vi "Modbus_建立连接.vi"(8 "error in (no error)":errorcluster caption="错误输入（无错误）", 10 "Mod ID":i32, 11 "Mod":T1) -> (0 "error out":errorcluster caption="错误输出", 3 "Mod 2":T1)   [LabVIEW 2018]
uses:
  <vilib>/Modbus/master/Modbus Master.lvclass
  C:/Program Files (x86)/National Instruments/LabVIEW 2018/vi.lib/Modbus/subvis/Modbus API/Modbus API.lvclass
  <vilib>/Modbus/subvis/Modbus API/Modbus API.lvclass/Modbus API.ctl
  <vilib>/Modbus/subvis/Transmission Data Unit (ADU)/Transmission Data Unit/Transmission Data Unit.lvclass/Transmission Data Unit.ctl
  <vilib>/Modbus/master/Data Access/Read Timeout/Set Read Timeout.vi
  <vilib>/Modbus/master/Data Access/Write Timeout/Set Write Timeout.vi
  <vilib>/Modbus/master/Data Access/Unit ID/Set Unit ID Property.vi
  <vilib>/Modbus/subvis/Modbus API/Read Transmission Data Unit.vi
  <vilib>/Modbus/subvis/Modbus API/Write Transmission Data Unit.vi
  <vilib>/Modbus/subvis/Transmission Data Unit (ADU)/Transmission Data Unit/Data Access/timeouts/Write read operation timeout.vi
  <vilib>/Modbus/subvis/Transmission Data Unit (ADU)/Transmission Data Unit/Data Access/timeouts/Write write operation timeout.vi
  <vilib>/Modbus/subvis/Transmission Data Unit (ADU)/Transmission Data Unit/Data Access/Unit ID/Write Unit ID.vi
  <vilib>/Modbus/master/Create Master Instance (Serial).vi
  <vilib>/Modbus/master/Create Master Instance (TCP).vi
  <vilib>/Modbus/subvis/Transmission Data Unit (ADU)/Transmission Data Unit/Transmission Data Unit.lvclass
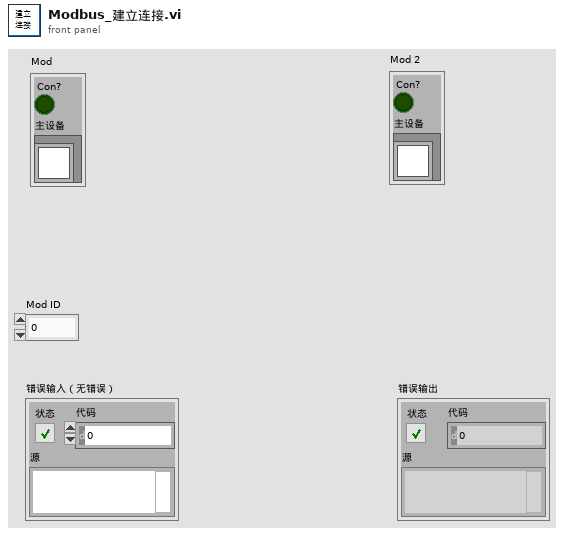
[diagram p1: front panel]
types:
  T1 = cluster{"Con?":bool, "主设备":refnum<class "Modbus Master.lvclass">}
  T2 = cluster{"设备站号":u8, "IP Addr":string, "Port":u16, "COM":string, "baud rate (9600)":u32, "Protocol":enum16{"Serial Port", "Modbus TCP/IP"}}
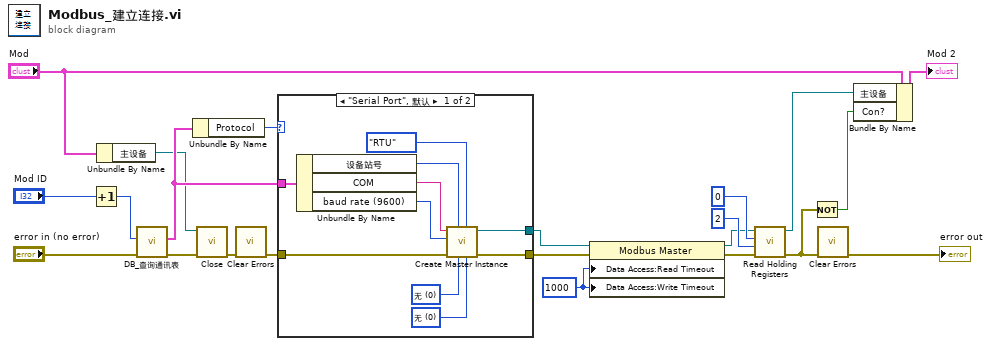
[diagram p0: block diagram]
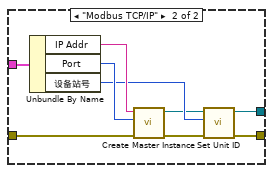
[diagram p2: hidden frame]
diagram:
  w9 = 1000 ("Write Timeout")
  n1 = Increment(x="Mod ID") -> (x+1=w20:i32)
  n2 = Unbundle By Name("Mod") -> ("主设备"=w16:refnum<class "Modbus Master.lvclass">)
  n3 = call "DB_查询通讯表.vi"("error in (no error)"="error in (no error)", "ID"=w20) -> ("error out"=w15:errorcluster, "设备通讯参数"=w18:T2)  [unwired: 8 in]
  n4 = Unbundle By Name(w18) -> ("Protocol"=w19:enum16{"Serial Port", "Modbus TCP/IP"})
  n5 = call-dynamic "Close.vi"("error in (no error)"=w15, "Modbus master in"=w16) -> ("error out"=w17:errorcluster)  [unwired: 9 in]
  n6 = call <vilib>:"Clear Errors.vi"("error in (no error)"=w17) -> ("error out"=w14:errorcluster)  [unwired: 5 in, 1 out]
  n7 = case shown="\"Serial Port\", 默认" w19 {
    tunnel: w14 -> [w29 w40]
    tunnel: w18 -> [w32 w41]
    tunnel: [w24 w33] -> w3
    tunnel: [w23 w34] -> w4
    frame "Serial Port", Default {
      w27 = u16 0 items=["无", "XON/XOFF", "RTS/CTS", "XON/XOFF & RTS/CTS", "DTR/DSR", "XON/XOFF & DTR/DSR"] ("flow control (None)")
      w28 = u16 0 items=["无", "奇", "偶"] ("parity (Even)")
      n8 = Unbundle By Name ("按名称解除捆绑")(w32) -> ("设备站号"=w26:u8, "COM"=w31:string, "baud rate (9600)"=w30:u32)
      n9 = call-poly <vilib>:"Create Master Instance.vi"("flow control (None)"=w27, "serial type"=enum16{"RTU", "ASCII"}."RTU", "parity (Even)"=w28, "unit ID"=w26, "error in (no error)"=w29, "baud rate (9600)"=w30, "VISA resource name"=w31) -> ("error out"=w23:errorcluster, "serial master instance"=w24:refnum<class "Modbus Master.lvclass">)  [unwired: 3 in]
    }
    frame "Modbus TCP/IP" {
      n10 = Unbundle By Name ("按名称解除捆绑")(w41) -> ("IP Addr"=w39:string, "Port"=w38:u16, "设备站号"=w37:u8)
      n11 = call-poly <vilib>:"Create Master Instance.vi"("error in (no error)"=w40, "port (502)"=w38, "address"=w39) -> ("error out"=w36:errorcluster, "TCP master instance"=w35:refnum<class "Modbus Master.lvclass">)  [unwired: 7 in]
      n12 = call <vilib>:"Set Unit ID.vi"("error in (no error)"=w36, "unit ID"=w37, "Modbus master in"=w35) -> ("error out"=w34:errorcluster, "Modbus master out"=w33:refnum<class "Modbus Master.lvclass">)  [unwired: 7 in]
    }
  }
  n13 = property on="属性节点" class="Modbus Master"(reference=w3, error in=w4, "Data Access:Read Timeout"=w9, "Data Access:Write Timeout"=w9) -> (reference out=w5:refnum<class "Modbus Master.lvclass">, error out=w6:errorcluster)
  n14 = call-dynamic "Read Holding Registers.vi"("error in (no error)"=w6, "number of holding registers"=u16 2 ("number of coils"), "starting address"=u16 0, "Modbus master in"=w5) -> ("error out"=w1:errorcluster, "Modbus master out"=w2:refnum<class "Modbus Master.lvclass">)  [unwired: 5 in, 1 out]
  n15 = Not(x=w1) -> (.not. x?=w10:bool)
  n16 = call <vilib>:"Clear Errors.vi"("error in (no error)"=w1) -> ("error out"=→"error out":errorcluster)  [unwired: 5 in, 1 out]
  n17 = Bundle By Name(cluster="Mod", "主设备"=w2, "Con?"=w10) -> (→"Mod 2":T1)
